vi "Safety_Check.vi"(1 "Adam Loop Count":i32, 2 "Ch Names":string[](array[string]), 3 "Values":dbl[](array[numeric]) format="%.2f") -> (0 "Scan comment":string)   [LabVIEW 2012]
uses:
  ADAM Client/Sub VIs/ADAM Controls/Update_scan_value.ctl
  Anemometry/Anemometry Sub Vis/Globals/Gas_management_global.vi
  ADAM_Global.vi
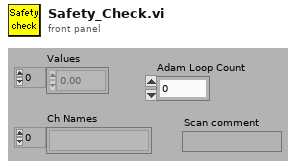
[diagram p1: front panel]
types:
  T1 = cluster{"Channel name":string, "Set value of A to":dbl, "Set value of B to":dbl, "Set value of C to":dbl, "Set value of D to":dbl}
  T2 = typedef "Update_scan_value.ctl" = cluster{"Channel Name":string, "New Value":dbl}
  T3 = enum16{"Append to Global", "Read Global then Clear"}
  T4 = enum16{"On", "Off", "Always On", "Always Off", "Delete"}
  T5 = typedef "LVDateTimeRec.ctl" = cluster{"fractional second":dbl, "second":i32, "minute":i32, "hour":i32, "day of month":i32, "month":i32, "year":i32, "day of week":i32, "day of year":i32, "DST":i32}
  T6 = cluster{"Channel name":string, "Set value of A to":dbl, "Set value of B to":dbl, "Set value of C to":dbl, "Set value of D to":dbl}[]
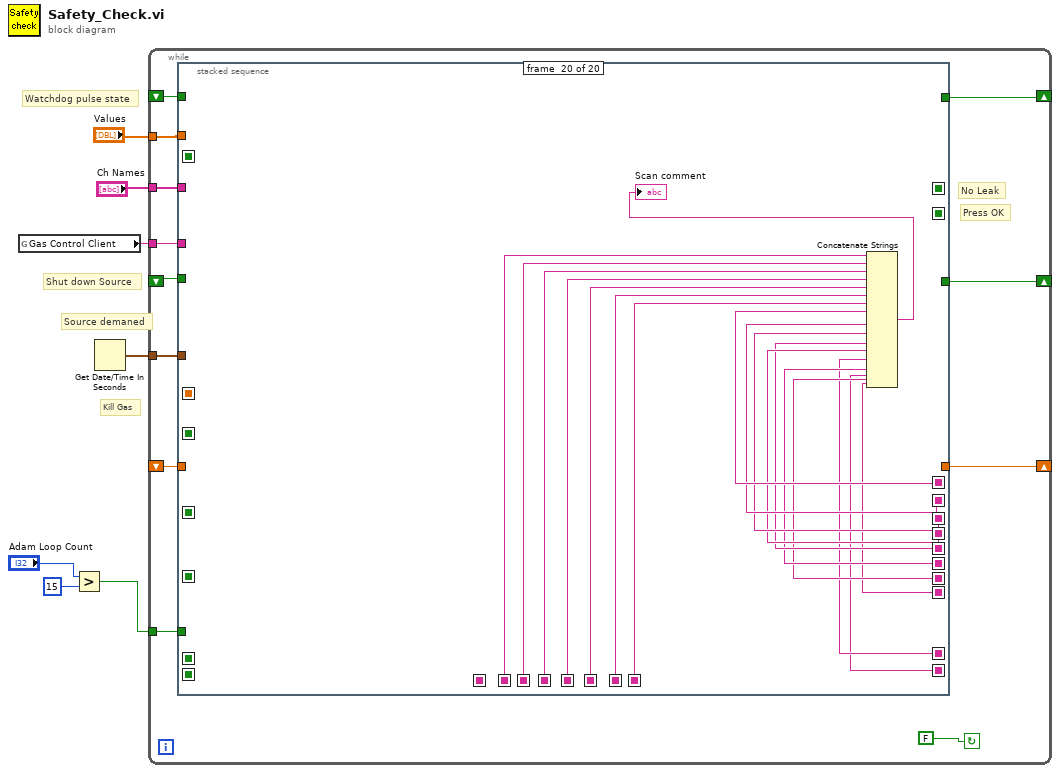
[diagram p0: block diagram]
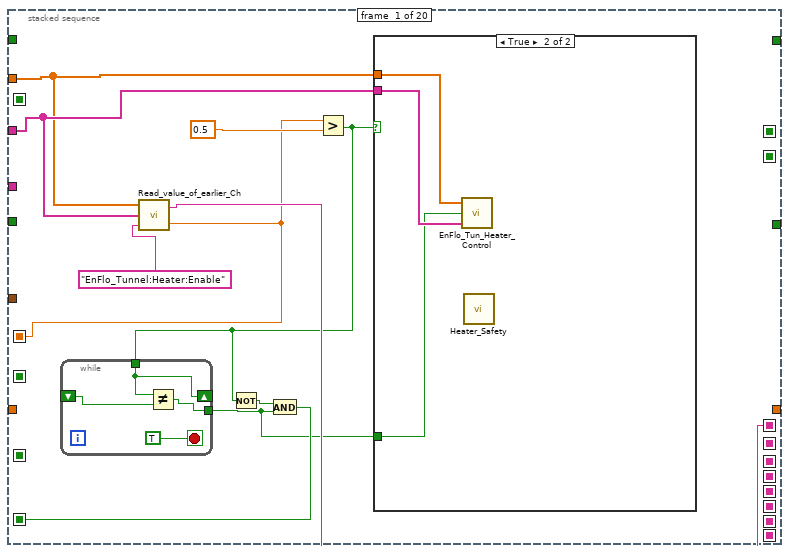
[diagram p2: hidden frame]
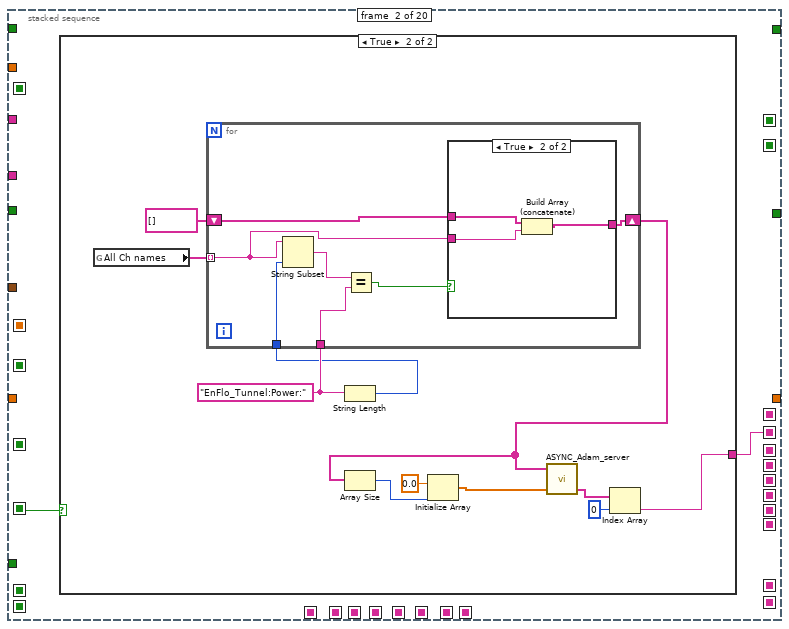
[diagram p4: hidden frame]
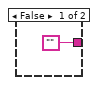
[diagram p5: hidden frame]
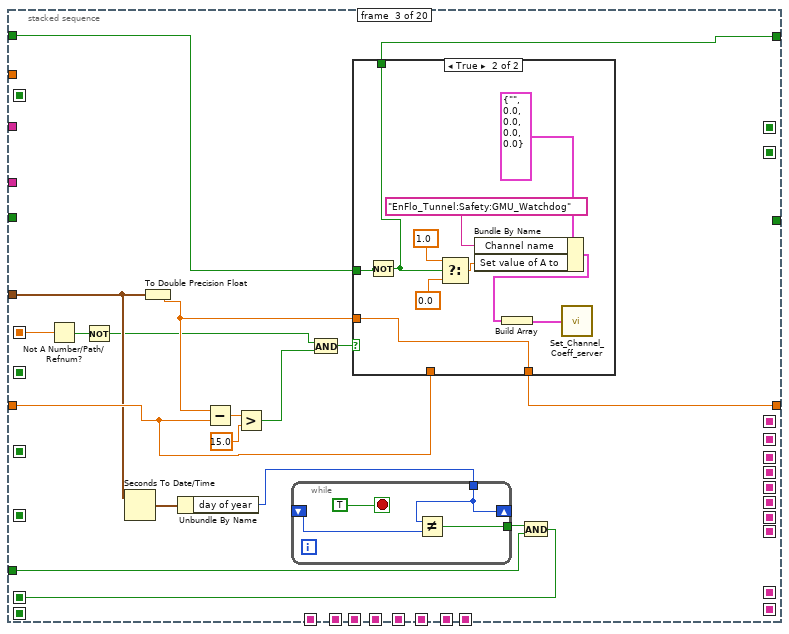
[diagram p7: hidden frame]
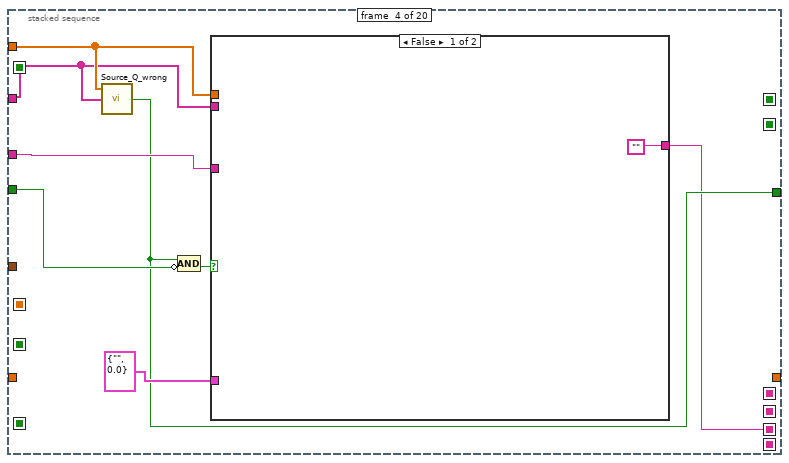
[diagram p9: hidden frame]
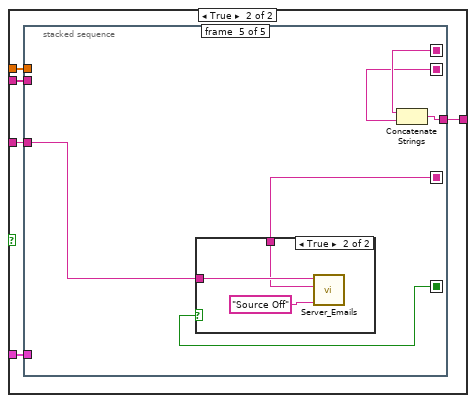
[diagram p10: hidden frame]
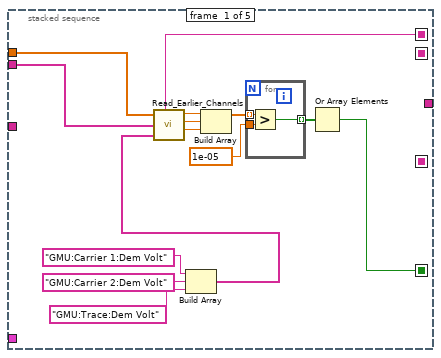
[diagram p11: hidden frame]
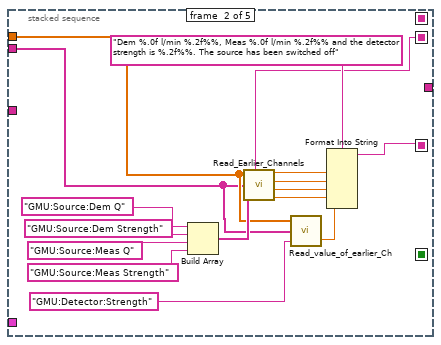
[diagram p12: hidden frame]
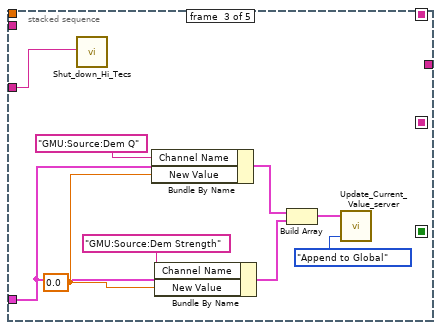
[diagram p13: hidden frame]
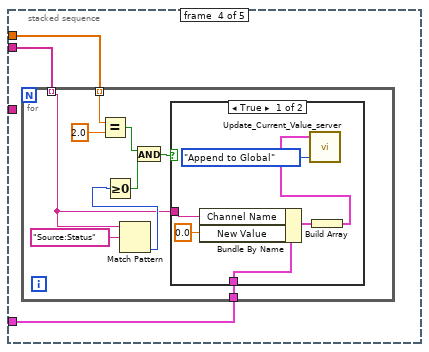
[diagram p14: hidden frame]
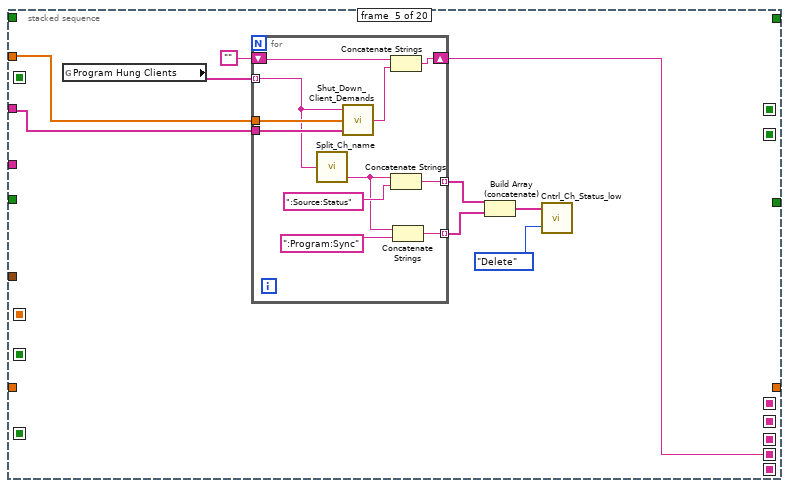
[diagram p17: hidden frame]
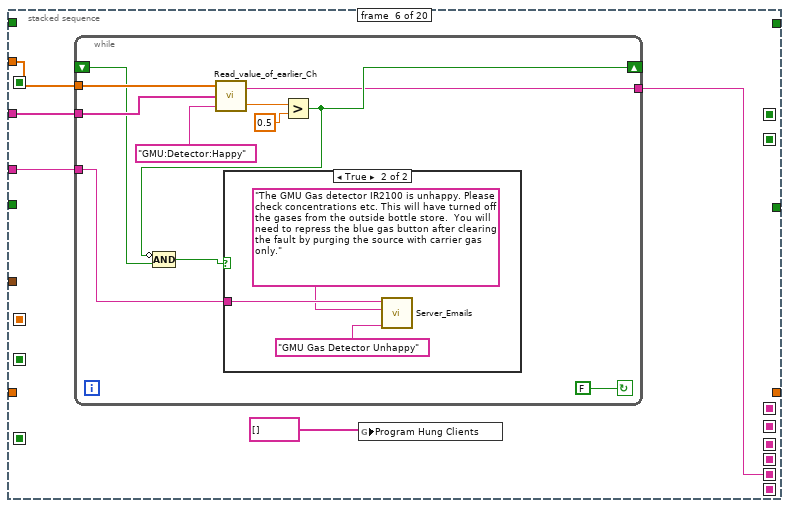
[diagram p18: hidden frame]
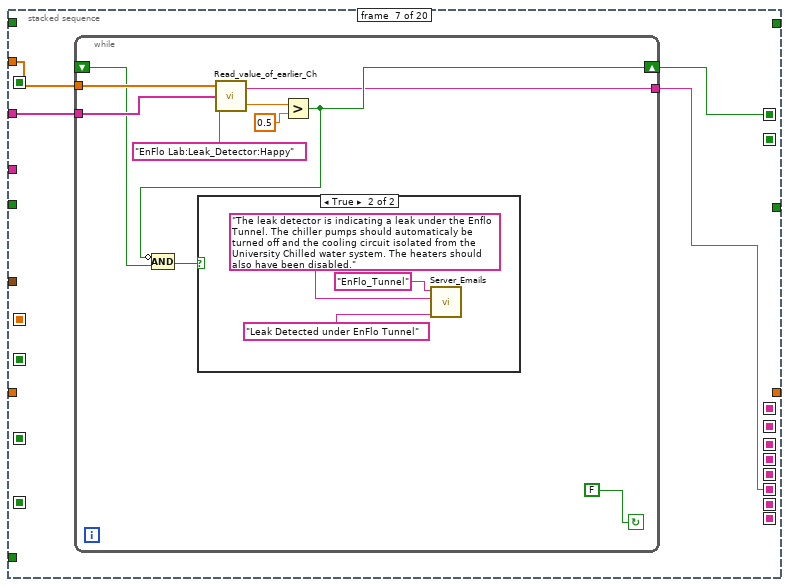
[diagram p20: hidden frame]
diagram:
  # "Shut down Source"
  # "Source demaned"
  # "Watchdog pulse state"
  # "Kill Gas"
  n1 = global read "Gas_management_global.vi" "Gas Control Client"() -> (w5:string)
  n2 = Greater?(x="Adam Loop Count", y=15) -> (0:w2:bool)
  n3 = Get Date/Time In Seconds() -> (seconds since 1Jan1904=w1:timestamp)
  n4 = while {
    shift-left: _ -> [w14]
    shift-right: [w13] -> _
    shift-left: _ -> [w16]
    shift-right: [w15] -> _
    tunnel: w5 -> [w18]
    tunnel: "Ch Names" -> [w19]
    tunnel: "Values" -> [w17]
    shift-right: [w11] -> _
    shift-left: _ -> [w10]
    tunnel: w2 -> [w9]
    tunnel: w1 -> [w8]
    stop <- FALSE continue-if-true
    # "Press OK"
    # "No Leak"
    n5 = stacked-sequence {
      seq-local: [_ _ _ _ _ _ w219 _ _ _ _ _ _ _ _ _ _ _ _ _] -> [_ _ _ _ _ _ _ _ _ _ _ _ w401 _ _ _ _ _ _ _]
      seq-local: [w22 _ _ _ _ _ _ _ _ _ _ _ _ _ _ _ _ _ _ _] -> [_ w38 _ _ _ _ _ _ _ _ _ _ _ _ _ _ _ _ _ _]
      seq-local: [_ _ w68 _ _ _ _ _ _ _ _ _ _ _ _ _ _ _ _ _] -> [_ _ _ _ _ _ _ _ _ _ _ _ _ _ _ _ _ _ _ _]
      seq-local: [_ _ _ _ _ _ _ _ _ _ _ _ _ _ w462 _ _ _ _ _] -> [_ _ _ _ _ _ _ _ _ _ _ _ _ _ _ w478 _ _ _ _]
      seq-local: [_ _ _ _ _ _ _ _ _ _ _ _ _ _ _ w470 _ _ _ _] -> [_ _ _ _ _ _ _ _ _ _ _ _ _ _ _ _ _ _ w602 _]
      seq-local: [w25 _ _ _ _ _ _ _ _ _ _ _ _ _ _ _ _ _ _ _] -> [_ _ _ _ _ _ _ _ _ _ _ _ _ _ _ _ _ _ _ w638]
      seq-local: [_ w37 _ _ _ _ _ _ _ _ _ _ _ _ _ _ _ _ _ _] -> [_ _ _ _ _ _ _ _ _ _ _ _ _ _ _ _ _ _ _ w637]
      seq-local: [_ _ _ w96 _ _ _ _ _ _ _ _ _ _ _ _ _ _ _ _] -> [_ _ _ _ _ _ _ _ _ _ _ _ _ _ _ _ _ _ _ w636]
      seq-local: [_ _ _ _ w179 _ _ _ _ _ _ _ _ _ _ _ _ _ _ _] -> [_ _ _ _ _ _ _ _ _ _ _ _ _ _ _ _ _ _ _ w635]
      seq-local: [_ _ _ _ _ w199 _ _ _ _ _ _ _ _ _ _ _ _ _ _] -> [_ _ _ _ _ _ _ _ _ _ _ _ _ _ _ _ _ _ _ w634]
      seq-local: [_ _ _ _ _ _ w218 _ _ _ _ _ _ _ _ _ _ _ _ _] -> [_ _ _ _ _ _ _ _ _ _ _ _ _ _ _ _ _ _ _ w633]
      seq-local: [_ _ _ _ _ _ _ _ _ w326 _ _ _ _ _ _ _ _ _ _] -> [_ _ _ _ _ _ _ _ _ _ _ _ _ _ _ _ _ _ _ w632]
      seq-local: [_ _ _ _ _ _ _ _ _ _ w358 _ _ _ _ _ _ _ _ _] -> [_ _ _ _ _ _ _ _ _ _ _ _ _ _ _ _ _ _ _ w623]
      seq-local: [_ _ _ _ _ _ _ _ _ _ _ w378 _ _ _ _ _ _ _ _] -> [_ _ _ _ _ _ _ _ _ _ _ _ _ _ _ _ _ _ _ w622]
      seq-local: [_ _ _ _ _ _ _ _ _ _ _ _ w402 _ _ _ _ _ _ _] -> [_ _ _ _ _ _ _ _ _ _ _ _ _ _ _ _ _ _ _ w625]
      seq-local: [_ _ _ _ _ _ _ _ _ _ _ _ _ w429 _ _ _ _ _ _] -> [_ _ _ _ _ _ _ _ _ _ _ _ _ _ _ _ _ _ _ w626]
      seq-local: [_ _ _ _ _ _ _ _ _ _ _ _ _ _ w453 _ _ _ _ _] -> [_ _ _ _ _ _ _ _ _ _ _ _ _ _ _ _ _ _ _ w627]
      seq-local: [_ _ _ _ _ _ _ _ _ _ _ _ _ _ _ w467 _ _ _ _] -> [_ _ _ _ _ _ _ _ _ _ _ _ _ _ _ _ _ _ _ w628]
      seq-local: [_ _ _ _ _ _ _ _ _ _ _ _ _ _ _ _ w535 _ _ _] -> [_ _ _ _ _ _ _ _ _ _ _ _ _ _ _ _ _ _ _ w629]
      seq-local: [_ _ _ _ _ _ _ _ _ _ _ _ _ _ _ _ _ w564 _ _] -> [_ _ _ _ _ _ _ _ _ _ _ _ _ _ _ _ _ _ _ w630]
      seq-local: [_ _ _ _ _ _ _ _ _ _ _ _ _ _ _ _ _ _ w600 _] -> [_ _ _ _ _ _ _ _ _ _ _ _ _ _ _ _ _ _ _ w631]
      seq-local: [w24 _ _ _ _ _ _ _ _ _ _ _ _ _ _ _ _ _ _ _] -> [_ _ w66 _ _ _ _ _ _ _ _ _ _ _ _ _ _ _ _ _]
      seq-local: [_ _ _ _ _ _ _ _ _ _ _ _ _ _ w452 _ _ _ _ _] -> [_ _ _ _ _ _ _ _ _ _ _ _ _ _ _ w466 _ _ _ _]
      seq-local: [_ _ _ _ _ _ _ w237 _ _ _ _ _ _ _ _ _ _ _ _] -> [_ _ _ _ _ _ _ _ _ _ _ _ w400 _ _ _ _ _ _ _]
      seq-local: [_ _ _ _ _ _ _ w236 _ _ _ _ _ _ _ _ _ _ _ _] -> [_ _ _ _ _ _ _ _ _ _ _ _ _ _ _ _ _ _ _ w621]
      seq-local: [_ _ _ _ _ _ _ w235 _ _ _ _ _ _ _ _ _ _ _ _] -> [_ _ _ _ _ _ _ _ w267 _ _ _ _ _ _ _ _ _ _ _]
      seq-local: [_ _ _ _ _ _ _ _ w264 _ _ _ _ _ _ _ _ _ _ _] -> [_ _ _ _ _ _ _ _ _ _ _ _ _ _ _ _ _ _ _ _]
      tunnel: w19 -> [w27 _ _ w98 w186 w201 w220 w238 w265 w327 w359 w380 w403 w435 w458 w479 w540 w567 _ _]
      tunnel: w18 -> [_ _ _ w103 _ w200 _ _ _ _ _ _ _ _ _ _ _ _ _ _]
      tunnel: w17 -> [w26 _ _ w99 w182 w202 w221 w239 w266 w328 w360 w381 w404 w436 w459 w480 w541 w568 _ _]
      tunnel: w16 -> [_ _ w79 _ _ _ _ _ _ _ _ _ _ _ _ _ _ _ _ _]
      tunnel: [_ _ w78 _ _ _ _ _ _ _ _ _ _ _ _ _ _ _ _ _] -> w15
      tunnel: w14 -> [_ _ _ w102 _ _ _ _ _ _ _ _ _ _ _ _ _ _ _ _]
      tunnel: [_ _ _ w97 _ _ _ _ _ _ _ _ _ _ _ _ _ _ _ _] -> w13
      tunnel: [_ _ w77 _ _ _ _ _ _ _ _ _ _ _ _ _ _ _ _ _] -> w11
      tunnel: w10 -> [_ _ w73 _ _ _ _ _ _ _ _ _ _ _ _ _ _ _ _ _]
      tunnel: w9 -> [_ _ w69 _ _ _ _ _ _ _ _ w379 _ _ _ w471 w536 _ w601 _]
      tunnel: w8 -> [_ _ w67 _ _ _ _ _ _ _ _ _ _ _ _ _ _ _ _ _]
      frame #0 {
        n6 = call "Read_value_of_earlier_Ch.vi"("Desired Ch to Read"="EnFlo_Tunnel:Heater:Enable", "Ch names"=w27, "Present scan array"=w26) -> ("Value"=w24:dbl, "Scan comment"=w25:string)  [unwired: 1 in]
        n7 = Greater?(x=w24, y=0.5) -> (0:w23:bool)
        n8 = while {
          shift-right: [w33] -> _
          shift-left: _ -> [w32]
          tunnel: w23 -> [w33]
          tunnel: [w30] -> w20
          stop <- TRUE stop-if-true
          n9 = Not Equal?(x=w33, y=w32) -> (x != y?=w30:bool)
        }
        n10 = Not(x=w23) -> (.not. x?=w21:bool)
        n11 = And(x=w21, y=w20) -> (x .and. y?=w22:bool)
        n12 = case shown="True" w23 {
          tunnel: w26 -> [_ w36]
          tunnel: w27 -> [_ w35]
          tunnel: w20 -> [_ w34]
          frame False {
          }
          frame True {
            n13 = call "EnFlo_Tun_Heater_Control.vi"("Ch Names"=w35, "Heaters Just Enabled"=w34, "Values"=w36) -> ()  [unwired: 1 in]
            n14 = call "Heater_Safety.vi"() -> ()  [unwired: 3 in, 5 out]
          }
        }
      }
      frame #1 {
        n15 = case shown="True" w38 {
          tunnel: ["" w41] -> w37
          frame False {
          }
          frame True {
            w50 = "EnFlo_Tunnel:Power:"
            n16 = global read "ADAM_Global.vi" "All Ch names"() -> (w40:string[])
            n17 = String Length(string=w50) -> (length=w49:i32)
            n18 = for {
              shift-right: [w52] -> w45
              shift-left: string[] [] -> [w53]
              tunnel: w40 -> [w56] mode=indexing
              tunnel: w49 -> [w57]
              tunnel: w50 -> [w54]
              n19 = String Subset(string=w56, length (rest)=w57) -> (substring=w55:string)  [unwired: 1 out]
              n20 = Equal?(x=w55, y=w54) -> (x = y?=w51:bool)
              n21 = case shown="True" w51 {
                tunnel: w56 -> [_ w61]
                tunnel: w53 -> [w58 w59]
                tunnel: [w58 w60] -> w52
                frame False {
                }
                frame True {
                  n22 = Build Array (concatenate)(w59, w61) -> (w60:string[])
                }
              }
            }
            n23 = Array Size(array=w45) -> (size(s)=w46:i32)
            n24 = Initialize Array(0.0 ("element"), w46) -> (w44:dbl[])
            n25 = call "ASYNC_Adam_server.vi"("Values"=w44, "Channel Names"=w45) -> ("Scan Comments"=w43:string[])  [unwired: 1 in, 2 out]
            n26 = Index Array(array=w43, index=0) -> (element=w41:string)
          }
        }
      }
      frame #2 {
        n27 = Not A Number/Path/Refnum?(number/path/refnum=w66) -> (NaN/Path/Refnum?=w65:bool)
        n28 = Not(x=w65) -> (.not. x?=w63:bool)
        n29 = Seconds To Date/Time(time stamp (now)=w67) -> (date time rec=w72:T5)  [unwired: 1 in]
        n30 = To Double Precision Float(number=w67) -> (double precision float=w76:dbl)
        n31 = Unbundle By Name(w72) -> ("day of year"=w71:i32)
        n32 = Subtract(x=w76, y=w73) -> (x-y=w75:dbl)
        n33 = Greater?(x=w75, y=15.0) -> (0:w64:bool)
        n34 = while {
          shift-right: [w83] -> _
          shift-left: _ -> [w82]
          tunnel: w71 -> [w83]
          tunnel: [w81] -> w70
          stop <- TRUE stop-if-true
          n35 = Not Equal?(x=w83, y=w82) -> (x != y?=w81:bool)
        }
        n36 = And(x=w63, y=w64) -> (x .and. y?=w62:bool)
        n37 = case shown="True" w62 {
          tunnel: w79 -> [w84 w88]
          tunnel: [w84 w87] -> w78
          tunnel: [w85 w86] -> w77
          tunnel: w76 -> [_ w86]
          tunnel: w73 -> [w85 _]
          frame False {
          }
          frame True {
            n38 = Not(x=w88) -> (.not. x?=w87:bool)
            n39 = Select(t=1.0 ("Suction"), s=w87, f=0.0 ("Suction")) -> (s? t:f=w91:dbl)
            n40 = Bundle By Name(cluster=T1 {"Channel name"="", "Set value of A to"=0.0, "Set value of B to"=0.0, "Set value of C to"=0.0, "Set value of D to"=0.0}, "Channel name"="EnFlo_Tunnel:Safety:GMU_Watchdog" ("Desired Ch to Read"), "Set value of A to"=w91) -> (w95:T1)
            n41 = Build Array(w95) -> (w90:T6)
            n42 = call "Set_Channel_Coeff_server.vi"("Set Array"=w90) -> ()
          }
        }
        n43 = And(x=w70, y=w69) -> (x .and. y?=w68:bool)
      }
      frame #3 {
        n44 = call "Source_Q_wrong.vi"("Ch Names"=w98, "Values"=w99) -> ("Gas Error?"=w97:bool)  [unwired: 1 out]
        n45 = Compound Arithmetic op=AND(w97, invert w102) -> (w101:bool)
        n46 = case shown="False" w101 {
          tunnel: w103 -> [_ w109]
          tunnel: w99 -> [_ w108]
          tunnel: w98 -> [_ w107]
          tunnel: T2 {"Channel Name"="", "New Value"=0.0} ("Update Scan Value Cluster") -> [_ w106]
          tunnel: ["" w105] -> w96
          frame False {
          }
          frame True {
            n47 = stacked-sequence {
              seq-local: [_ w141 _ _ _] -> [_ _ _ _ w174]
              seq-local: [w111 _ _ _ _] -> [_ _ _ _ w173]
              seq-local: [w110 _ _ _ _] -> [_ _ _ _ w172]
              seq-local: [_ w127 _ _ _] -> [_ _ _ _ w171]
              tunnel: w109 -> [_ _ w144 _ w175]
              tunnel: w108 -> [w121 w131 _ w153 _]
              tunnel: w107 -> [w122 w130 _ w154 _]
              tunnel: w106 -> [_ _ w143 w152 _]
              tunnel: [_ _ _ _ w170] -> w105
              frame #0 {
                n48 = Build Array("GMU:Carrier 1:Dem Volt", "GMU:Carrier 2:Dem Volt", "GMU:Trace:Dem Volt") -> (w123:string[])
                n49 = call "Read_Earlier_Channels.vi"("Present scan array"=w121, "Ch names"=w122, "Desired Channels"=w123) -> ("Scan comments"=w110:string, "Index 0"=w117:dbl, "Index 1"=w116:dbl, "Index 2"=w115:dbl)  [unwired: 2 out]
                n50 = Build Array(w117, w116, w115) -> (w114:dbl[])
                n51 = for {
                  tunnel: w114 -> [w126] mode=indexing
                  tunnel: 1e-05 -> [w125]
                  tunnel: [w124] -> w112 mode=indexing
                  n52 = Greater?(x=w126, y=w125) -> (0:w124:bool)
                }
                n53 = Or Array Elements(Boolean array=w112) -> (logical OR=w111:bool)
              }
              frame #1 {
                n54 = Build Array("GMU:Source:Dem Q", "GMU:Source:Dem Strength", "GMU:Source:Meas Q", "GMU:Source:Meas Strength") -> (w136:string[])
                n55 = call "Read_Earlier_Channels.vi"("Present scan array"=w131, "Ch names"=w130, "Desired Channels"=w136) -> ("Scan comments"=w127:string, "Index 0"=w135:dbl, "Index 1"=w134:dbl, "Index 2"=w133:dbl, "Index 3"=w132:dbl)  [unwired: 1 out]
                n56 = call "Read_value_of_earlier_Ch.vi"("Desired Ch to Read"="GMU:Detector:Strength", "Ch names"=w130, "Present scan array"=w131) -> ("Value"=w128:dbl)  [unwired: 1 in, 1 out]
                n57 = Format Into String(format string="Dem %.0f l/min %.2f%%, Meas %.0f l/min %.2f%% and the detector strength is %.2f%%. The source has been switched off" ("Format String"), w135, w134, w133, w132, w128) -> (resulting string=w141:string)  [unwired: 2 in, 1 out]
              }
              frame #2 {
                w145 = 0.0 ("Bundle Element")
                n58 = call "Shut_down_Hi_Tecs.vi"("Client Name"=w144) -> ()  [unwired: 6 out]
                n59 = Bundle By Name(cluster=w143, "Channel Name"="GMU:Source:Dem Q", "New Value"=w145) -> (w150:T2)
                n60 = Bundle By Name(cluster=w143, "Channel Name"="GMU:Source:Dem Strength", "New Value"=w145) -> (w151:T2)
                n61 = Build Array(w150, w151) -> (w147:T2[])
                n62 = call "Update_Current_Value_server.vi"("Mode"=T3."Append to Global", "Update array in"=w147) -> ()  [unwired: 1 in, 1 out]
              }
              frame #3 {
                n63 = for {
                  tunnel: w154 -> [w155] mode=indexing
                  tunnel: w153 -> [w161] mode=indexing
                  tunnel: w152 -> [w156]
                  n64 = Equal?(x=w161, y=2.0) -> (x = y?=w158:bool)
                  n65 = Match Pattern(string=w155, regular expression="Source:Status") -> (offset past match=w162:i32)  [unwired: 4 out]
                  n66 = Greater Or Equal To 0?(x=w162) -> (x >= 0?=w159:bool)
                  n67 = And(x=w158, y=w159) -> (x .and. y?=w157:bool)
                  n68 = case shown="True" w157 {
                    tunnel: w156 -> [w169 _]
                    tunnel: w155 -> [w168 _]
                    frame True {
                      n69 = Bundle By Name(cluster=w169, "Channel Name"=w168, "New Value"=0.0) -> (w166:T2)
                      n70 = Build Array(w166) -> (w165:T2[])
                      n71 = call "Update_Current_Value_server.vi"("Mode"=T3."Append to Global", "Update array in"=w165) -> ()  [unwired: 1 in, 1 out]
                    }
                    frame False {
                    }
                  }
                }
              }
              frame #4 {
                n72 = case shown="True" w173 {
                  tunnel: w175 -> [_ w178]
                  tunnel: w174 -> [_ w177]
                  frame False {
                  }
                  frame True {
                    n73 = call "Server_Emails.vi"("Client Name Contains"=w178, "Message"=w177, "Subject"="Source Off") -> ()  [unwired: 2 in, 3 out]
                  }
                }
                n74 = Concatenate Strings(w172, w171) -> (w170:string)
              }
            }
          }
        }
      }
      frame #4 {
        n75 = global read "ADAM_Global.vi" "Program Hung Clients"() -> (w187:string[])
        n76 = for {
          tunnel: w187 -> [w196] mode=indexing
          tunnel: w182 -> [w198]
          tunnel: w186 -> [w197]
          tunnel: [w194] -> w185 mode=indexing
          tunnel: [w191] -> w184 mode=indexing
          shift-right: [w189] -> w179
          shift-left: "" -> [w190]
          n77 = call "Split_Ch_name.vi"("Ch name"=w196) -> ("Low level"=w193:string)  [unwired: 2 out]
          n78 = call "Shut_Down_Client_Demands.vi"("Ch Names"=w197, "Values"=w198, "Client Name"=w196) -> ("Comments"=w188:string)
          n79 = Concatenate Strings(w190, w188) -> (w189:string)
          n80 = Concatenate Strings(w193, ":Source:Status") -> (w194:string)
          n81 = Concatenate Strings(w193, ":Program:Sync") -> (w191:string)
        }
        n82 = Build Array (concatenate)(w185, w184) -> (w183:string[])
        n83 = call "Cntrl_Ch_Status_low.vi"("Mode"=T4."Delete", "Channel names"=w183) -> ()  [unwired: 1 out]
      }
      frame #5 {
        n84 = while {
          tunnel: w202 -> [w214]
          tunnel: w201 -> [w213]
          shift-right: [w208] -> _
          shift-left: _ -> [w209]
          tunnel: w200 -> [w206]
          tunnel: [w204] -> w199
          stop <- FALSE continue-if-true
          n85 = call "Read_value_of_earlier_Ch.vi"("Desired Ch to Read"="GMU:Detector:Happy", "Ch names"=w213, "Present scan array"=w214) -> ("Value"=w211:dbl, "Scan comment"=w204:string)  [unwired: 1 in]
          n86 = Greater?(x=w211, y=0.5) -> (0:w208:bool)
          n87 = Compound Arithmetic op=AND(invert w208, w209) -> (w207:bool)
          n88 = case shown="True" w207 {
            tunnel: w206 -> [_ w216]
            frame False {
            }
            frame True {
              n89 = call "Server_Emails.vi"("Client Name Contains"=w216, "Message"="The GMU Gas detector IR2100 is unhappy. Please check concentrations etc. This will have turned off the gases from the outside bottle store.  You will need to repress the blue gas button after clearing the fault by purging the source with carrier gas only.", "Subject"="GMU Gas Detector Unhappy") -> ()  [unwired: 2 in, 3 out]
            }
          }
        }
        n90 = global write "ADAM_Global.vi" "Program Hung Clients"(string[] [] ("Program Hung Clients")) -> ()
      }
      frame #6 {
        n91 = while {
          tunnel: w221 -> [w231]
          tunnel: w220 -> [w230]
          shift-right: [w225] -> w219
          shift-left: _ -> [w226]
          tunnel: [w222] -> w218
          stop <- FALSE continue-if-true
          n92 = call "Read_value_of_earlier_Ch.vi"("Desired Ch to Read"="EnFlo Lab:Leak_Detector:Happy", "Ch names"=w230, "Present scan array"=w231) -> ("Value"=w228:dbl, "Scan comment"=w222:string)  [unwired: 1 in]
          n93 = Greater?(x=w228, y=0.5) -> (0:w225:bool)
          n94 = Compound Arithmetic op=AND(invert w225, w226) -> (w224:bool)
          n95 = case shown="True" w224 {
            frame False {
            }
            frame True {
              n96 = call "Server_Emails.vi"("Client Name Contains"="EnFlo_Tunnel", "Message"="The leak detector is indicating a leak under the Enflo Tunnel. The chiller pumps should automaticaly be turned off and the cooling circuit isolated from the  University Chilled water system. The heaters should also have been disabled.", "Subject"="Leak Detected under EnFlo Tunnel") -> ()  [unwired: 2 in, 3 out]
            }
          }
        }
      }
      frame #7 {
        n97 = while {
          tunnel: w239 -> [w245]
          tunnel: w238 -> [w244]
          shift-right: [w256] -> w237
          shift-left: _ -> [w257]
          tunnel: [w248] -> w236
          tunnel: [w240] -> w235
          stop <- FALSE continue-if-true
          n98 = call "Read_value_of_earlier_Ch.vi"("Desired Ch to Read"="EnFlo_Tunnel:Chiller_Pump:Enable", "Ch names"=w244, "Present scan array"=w245) -> ("Value"=w251:dbl, "Scan comment"=w249:string)  [unwired: 1 in]
          n99 = call "Read_value_of_earlier_Ch.vi"("Desired Ch to Read"="EnFlo_Tunnel:Chilled Water:Pressure_OK", "Ch names"=w244, "Present scan array"=w245) -> ("Value"=w259:dbl, "Scan comment"=w250:string)  [unwired: 1 in]
          n100 = call "Read_value_of_earlier_Ch.vi"("Desired Ch to Read"="EnFlo_Tunnel:Chiller_Pump:Running", "Ch names"=w244, "Present scan array"=w245) -> ("Value"=w242:dbl, "Scan comment"=w241:string)  [unwired: 1 in]
          n101 = Greater?(x=w259, y=0.5) -> (0:w256:bool)
          n102 = Greater?(x=w251, y=0.5) -> (0:w247:bool)
          n103 = Compound Arithmetic op=AND(invert w256, w257, w247) -> (w255:bool)
          n104 = case shown="True" w255 {
            frame False {
            }
            frame True {
              n105 = call "Server_Emails.vi"("Client Name Contains"="EnFlo_Tunnel", "Message"="The pressure in the chilled water  for the Enflo Tunnel has tripped the system. The chiller pumps should automaticaly be turned off and the cooling circuit isolated from the  University Chilled water system. The heaters should also have been disabled.", "Subject"="EnFlo Chilled Water Overpressure Trip") -> ()  [unwired: 2 in, 3 out]
            }
          }
          n106 = Greater?(x=w242, y=0.5) -> (0:w240:bool)
          n107 = Concatenate Strings(w249, w250, w241) -> (w248:string)
        }
      }
      frame #8 {
        n108 = case shown="True" w267 {
          tunnel: w266 -> [_ w296]
          tunnel: w265 -> [_ w295]
          tunnel: ["" w269] -> w264
          frame False {
          }
          frame True {
            w274 = "EnFlo_Tunnel:Chilled Water:Motor_Dem_Voltage"
            # "EnFlo_Tunnel:Chiller_Pump:Running"
            n109 = call "Read_value_of_earlier_Ch.vi"("Desired Ch to Read"="EnFlo_Tunnel:Chilled Water:Pressure_supply (Bar)", "Ch names"=w295, "Present scan array"=w296) -> ("Value"=w281:dbl, "Scan comment"=w273:string)  [unwired: 1 in]
            n110 = call "Read_value_of_earlier_Ch.vi"("Desired Ch to Read"="EnFlo_Tunnel:Chilled Water:Pressure_return (Bar)", "Ch names"=w295, "Present scan array"=w296) -> ("Value"=w291:dbl, "Scan comment"=w272:string)  [unwired: 1 in]
            n111 = call "Read_value_of_earlier_Ch.vi"("Desired Ch to Read"="EnFlo_Tunnel:Chilled Water:Desired_Delta_P", "Ch names"=w295, "Present scan array"=w296) -> ("Value"=w289:dbl, "Scan comment"=w271:string)  [unwired: 1 in]
            n112 = call "Read_value_of_earlier_Ch.vi"("Desired Ch to Read"=w274, "Ch names"=w295, "Present scan array"=w296) -> ("Value"=w279:dbl, "Scan comment"=w270:string)  [unwired: 1 in]
            n113 = Subtract(x=w281, y=w291) -> (x-y=w290:dbl)
            n114 = Subtract(x=w290, y=w289) -> (x-y=w277:dbl)
            n115 = Concatenate Strings(w273, w272, w271, w270) -> (w269:string)
            n116 = In Range and Coerce(upper limit=0.1 ("lower limit"), x=w277, lower limit=-0.1) -> (In Range?=w284:bool)  [unwired: 1 out]
            n117 = Less?(x=w281, y=3.9) -> (x < y?=w285:bool)
            n118 = Select(t=w284, s=w285, f=TRUE) -> (s? t:f=w278:bool)
            n119 = Less?(x=w281, y=4.0) -> (x < y?=w280:bool)
            n120 = case shown="True" w280 {
              tunnel: w279 -> [w307 w310]
              tunnel: w278 -> [_ w312]
              tunnel: w277 -> [_ w311]
              tunnel: [TRUE w309] -> w276
              tunnel: [w304 w308] -> w275
              frame False {
                n121 = Subtract(x=w307, y=0.2) -> (x-y=w304:dbl)
              }
              frame True {
                n122 = case shown="False" w312 {
                  tunnel: w311 -> [w317 _]
                  tunnel: w310 -> [w316 w324]
                  tunnel: [TRUE FALSE] -> w309
                  tunnel: [w314 w324] -> w308
                  frame False {
                    n123 = Greater Than 0?(x=w317) -> (x > 0?=w315:bool)
                    n124 = case shown="False" w315 {
                      tunnel: w316 -> [w319 w322]
                      tunnel: [w318 w321] -> w314
                      frame True {
                        n125 = Subtract(x=w319, y=0.1) -> (x-y=w318:dbl)
                      }
                      frame False {
                        n126 = Add(x=w322, y=0.1) -> (x+y=w321:dbl)
                      }
                    }
                  }
                  frame True {
                  }
                }
              }
            }
            n127 = case shown="True" w276 {
              tunnel: w275 -> [_ w298]
              tunnel: w274 -> [_ w301]
              frame False {
              }
              frame True {
                n128 = In Range and Coerce(upper limit=10.0, x=w298, lower limit=0.0) -> (coerced(x)=w297:dbl)  [unwired: 1 out]
                n129 = Build Array(w301) -> (w302:string[])
                n130 = Build Array(w297) -> (w303:dbl[])
                n131 = call "ASYNC_Adam_server.vi"("Values"=w303, "Channel Names"=w302) -> ()  [unwired: 1 in, 3 out]
              }
            }
          }
        }
      }
      frame #9 {
        n132 = while {
          tunnel: w328 -> [w344]
          tunnel: w327 -> [w343]
          shift-right: [w337] -> _
          shift-left: _ -> [w333]
          tunnel: [w329] -> w326
          stop <- FALSE continue-if-true
          w335 = 60.0 ("y")
          n133 = Decrement(x=w335) -> (x-1=w336:dbl)
          n134 = Select(t=w336, s=w333, f=w335) -> (s? t:f=w334:dbl)
          n135 = call "Read_value_of_earlier_Ch.vi"("Desired Ch to Read"="EnFlo_Tunnel:Chilled Water:Motor1 Temp", "Ch names"=w343, "Present scan array"=w344) -> ("Value"=w351:dbl, "Scan comment"=w331:string)  [unwired: 1 in]
          n136 = call "Read_value_of_earlier_Ch.vi"("Desired Ch to Read"="EnFlo_Tunnel:Chilled Water:Motor2 Temp", "Ch names"=w343, "Present scan array"=w344) -> ("Value"=w348:dbl, "Scan comment"=w330:string)  [unwired: 1 in]
          n137 = Greater?(x=w351, y=w334) -> (0:w345:bool)
          n138 = Greater?(x=w348, y=w334) -> (0:w346:bool)
          n139 = Or(x=w345, y=w346) -> (x .or. y?=w339:bool)
          n140 = call "Read_value_of_earlier_Ch.vi"("Desired Ch to Read"="EnFlo_Tunnel:Chiller_Pump:Enable", "Ch names"=w343, "Present scan array"=w344) -> ("Value"=w341:dbl, "Scan comment"=w332:string)  [unwired: 1 in]
          n141 = Greater?(x=w341, y=0.5) -> (0:w338:bool)
          n142 = And(x=w338, y=w339) -> (x .and. y?=w337:bool)
          n143 = Compound Arithmetic op=AND(w337, invert w333) -> (w350:bool)
          n144 = case shown="False" w350 {
            tunnel: w335 -> [_ w354]
            frame False {
            }
            frame True {
              n145 = Format Into String(format string="The Chilled Water Motor Temp is greater than %.0f deg C." ("Message"), w354) -> (resulting string=w353:string)  [unwired: 2 in, 1 out]
              n146 = call "Server_Emails.vi"("Client Name Contains"="EnFlo_Tunnel", "Message"=w353, "Subject"="Chilled Water Motor Temp") -> ()  [unwired: 2 in, 3 out]
            }
          }
          n147 = Concatenate Strings(w332, w331, w330) -> (w329:string)
        }
      }
      frame #10 {
        n148 = while {
          tunnel: w360 -> [w374]
          tunnel: w359 -> [w373]
          shift-right: [w362] -> _
          shift-left: _ -> [w368]
          shift-left: _ -> [w367]
          shift-left: _ -> [w366]
          tunnel: [w361] -> w358
          stop <- FALSE continue-if-true
          n149 = call "Read_value_of_earlier_Ch.vi"("Desired Ch to Read"="FFID:System:Enable", "Ch names"=w373, "Present scan array"=w374) -> ("Value"=w369:dbl, "Scan comment"=w361:string)  [unwired: 1 in]
          n150 = Greater?(x=w369, y=0.5) -> (0:w362:bool)
          n151 = Compound Arithmetic op=AND(w362, w368, invert w367, invert w366) -> (w364:bool)
          n152 = Compound Arithmetic op=AND(invert w362, invert w368, w367, w366) -> (w365:bool)
          n153 = Or(x=w364, y=w365) -> (x .or. y?=w363:bool)
          n154 = case shown="True" w363 {
            tunnel: w369 -> [_ w375]
            tunnel: w362 -> [_ _]
            frame False {
            }
            frame True {
              n155 = Build Array(w375) -> (w377:dbl[])
              n156 = call "ASYNC_Adam_server.vi"("Values"=w377, "Channel Names"=string[] ["GMU:Gas:Enable"]) -> ()  [unwired: 1 in, 3 out]
            }
          }
        }
      }
      frame #11 {
        # "Resetting A Tunnel speed to zero if the drive in turned off\nso that the belts do not slip when the tunnel is turned on again."
        n157 = while {
          tunnel: w381 -> [w394]
          tunnel: w380 -> [w393]
          shift-right: [w385] -> _
          shift-left: _ -> [w388]
          shift-left: _ -> [w387]
          shift-left: _ -> [w386]
          tunnel: w379 -> [w384]
          tunnel: [w382] -> w378
          stop <- FALSE continue-if-true
          n158 = call "Read_value_of_earlier_Ch.vi"("Desired Ch to Read"="A_Tunnel:Motor:Enable", "Ch names"=w393, "Present scan array"=w394) -> ("Value"=w389:dbl, "Scan comment"=w382:string)  [unwired: 1 in]
          n159 = Less?(x=w389, y=0.5) -> (x < y?=w385:bool)
          n160 = Compound Arithmetic op=AND(w385, w388, invert w387, invert w386, w384) -> (w383:bool)
          n161 = case shown="True" w383 {
            tunnel: w385 -> [_ _]
            frame False {
            }
            frame True {
              w397 = string[] ["A_Tunnel:Speed:Dem Velocity", "A_Tunnel:Speed:Dem Voltage"] ("Channel Names")
              n162 = Array Size(array=w397) -> (size(s)=w398:i32)
              n163 = Initialize Array(0.0 ("element"), w398) -> (w396:dbl[])
              n164 = call "ASYNC_Adam_server.vi"("Values"=w396, "Channel Names"=w397) -> ()  [unwired: 1 in, 3 out]
            }
          }
        }
      }
      frame #12 {
        n165 = And(x=w400, y=w401) -> (x .and. y?=w399:bool)
        n166 = case shown="False" w399 {
          tunnel: w404 -> [w409 _]
          tunnel: w403 -> [w408 _]
          tunnel: [w405 ""] -> w402
          frame False {
            n167 = for {
              tunnel: w409 -> [w419]
              tunnel: w408 -> [w418]
              tunnel: string[] ["EnFlo_Tunnel:Heater:Enable", "EnFlo_Tunnel:Chiller_Pump:Enable", "EnFlo_Tunnel:Tap_Water:Enable"] ("Ch Names") -> [w414] mode=indexing
              shift-right: [w412] -> w405
              shift-left: "" -> [w413]
              n168 = call "Read_value_of_earlier_Ch.vi"("Desired Ch to Read"=w414, "Ch names"=w418, "Present scan array"=w419) -> ("Value"=w416:dbl, "Scan comment"=w411:string)  [unwired: 1 in]
              n169 = Greater?(x=w416, y=0.5) -> (0:w415:bool)
              n170 = case shown="True" w415 {
                tunnel: w414 -> [_ w424]
                tunnel: ["" w421] -> w410
                frame False {
                }
                frame True {
                  n171 = Build Array(w424) -> (w427:string[])
                  n172 = Build Array(0.0) -> (w426:dbl[])
                  n173 = call "ASYNC_Adam_server.vi"("Values"=w426, "Channel Names"=w427) -> ("Scan Comments"=w422:string[])  [unwired: 1 in, 2 out]
                  n174 = Index Array(array=w422, index=0) -> (element=w421:string)
                }
              }
              n175 = Concatenate Strings(w413, w411, w410) -> (w412:string)
            }
          }
          frame True {
          }
        }
      }
      frame #13 {
        w437 = "EnFlo_Tunnel:Heater:Enable" ("Ch Name")
        n176 = call "Read_value_of_earlier_Ch.vi"("Desired Ch to Read"=w437, "Ch names"=w435, "Present scan array"=w436) -> ("Value"=w442:dbl, "Scan comment"=w431:string)  [unwired: 1 in]
        n177 = call "Read_value_of_earlier_Ch.vi"("Desired Ch to Read"="EnFlo_Tunnel:Reference:Velocity", "Ch names"=w435, "Present scan array"=w436) -> ("Value"=w439:dbl, "Scan comment"=w430:string)  [unwired: 1 in]
        n178 = Greater?(x=w442, y=0.5) -> (0:w434:bool)
        n179 = Less?(x=w439, y=0.25) -> (x < y?=w438:bool)
        n180 = And(x=w434, y=w438) -> (x .and. y?=w433:bool)
        n181 = case shown="True" w433 {
          tunnel: w437 -> [_ w448]
          tunnel: ["" w445] -> w432
          frame False {
          }
          frame True {
            n182 = Build Array(w448) -> (w451:string[])
            n183 = Build Array(0.0) -> (w450:dbl[])
            n184 = call "ASYNC_Adam_server.vi"("Values"=w450, "Channel Names"=w451) -> ("Scan Comments"=w446:string[])  [unwired: 1 in, 2 out]
            n185 = Index Array(array=w446, index=0) -> (element=w445:string)
          }
        }
        n186 = Concatenate Strings(w431, w430, w432) -> (w429:string)
      }
      frame #14 {
        n187 = call "Read_value_of_earlier_Ch.vi"("Desired Ch to Read"="EnFlo_Tunnel:Chiller_Pump:Running", "Ch names"=w458, "Present scan array"=w459) -> ("Value"=w460:dbl, "Scan comment"=w455:string)  [unwired: 1 in]
        n188 = call "Read_value_of_earlier_Ch.vi"("Desired Ch to Read"="EnFlo_Tunnel:Reference:Velocity", "Ch names"=w458, "Present scan array"=w459) -> ("Value"=w456:dbl, "Scan comment"=w454:string)  [unwired: 1 in]
        n189 = Greater?(x=w456, y=0.4) -> (0:w464:bool)
        n190 = Greater?(x=w460, y=0.5) -> (0:w452:bool)
        n191 = Compound Arithmetic op=AND(w452, w464) -> (w462:bool)
        n192 = Concatenate Strings(w455, w454) -> (w453:string)
      }
      frame #15 {
        w476 = "EnFlo_Tunnel:Heat_Ex_Div_Valve:Dem Pos"
        n193 = case shown="True" w478 {
          tunnel: w480 -> [_ w518]
          tunnel: w479 -> [_ w519]
          tunnel: w476 -> [_ w522]
          tunnel: [0.0 ("upper limit") w528] -> w472
          tunnel: ["" w513] -> w469
          frame False {
          }
          frame True {
            n194 = call "Read_value_of_earlier_Ch.vi"("Desired Ch to Read"="EnFlo_Tunnel:Exit Duct:Dem Temp", "Ch names"=w519, "Present scan array"=w518) -> ("Value"=w527:dbl, "Scan comment"=w517:string)  [unwired: 1 in]
            n195 = call "Read_value_of_earlier_Ch.vi"("Desired Ch to Read"="EnFlo_Tunnel:Exit Duct Top:Temp", "Ch names"=w519, "Present scan array"=w518) -> ("Value"=w523:dbl, "Scan comment"=w516:string)  [unwired: 1 in]
            n196 = call "Read_value_of_earlier_Ch.vi"("Desired Ch to Read"="EnFlo_Tunnel:Exit Duct:Temp", "Ch names"=w519, "Present scan array"=w518) -> ("Value"=w524:dbl, "Scan comment"=w515:string)  [unwired: 1 in]
            n197 = call "Read_value_of_earlier_Ch.vi"("Desired Ch to Read"=w522, "Ch names"=w519, "Present scan array"=w518) -> ("Value"=w525:dbl, "Scan comment"=w514:string)  [unwired: 1 in]
            n198 = Add(x=w523, y=w524) -> (x+y=w532:dbl)
            n199 = Divide(x=w532, y=2.0) -> (x/y=w534:dbl)
            n200 = Concatenate Strings(w517, w516, w515, w514) -> (w513:string)
            n201 = call "Back_End_Chiller_PID.vi"("Present Value"=w534, "Previous Control Sum"=w525, "Setpoint"=w527) -> ("Dem Output"=w531:dbl)
            n202 = In Range and Coerce(upper limit=100.0, x=w531, lower limit=0.0) -> (coerced(x)=w528:dbl)  [unwired: 1 out]
          }
        }
        n203 = while {
          shift-right: [w510] -> w477
          shift-left: _ -> [_]
          tunnel: w466 -> [w510]
          shift-left: _ -> [_]
          shift-left: _ -> [_]
          shift-left: _ -> [_]
          shift-left: _ -> [_]
          shift-left: _ -> [_]
          shift-left: _ -> [_]
          shift-left: _ -> [_]
          shift-left: _ -> [_]
          shift-left: _ -> [_]
          shift-left: _ -> [_]
          shift-left: _ -> [_]
          shift-left: _ -> [_]
          shift-left: _ -> [_]
          shift-left: _ -> [_]
          shift-left: _ -> [_]
          shift-left: _ -> [_]
          shift-left: _ -> [w509]
          tunnel: [w509] -> w475
          stop <- TRUE stop-if-true
        }
        n204 = And(x=w477, y=w475) -> (x .and. y?=w474:bool)
        n205 = case shown="False" w474 {
          tunnel: [w482 w493] -> w473
          tunnel: w472 -> [_ w493]
          tunnel: [w481 FALSE] -> w470
          frame False {
            # "Exercise valve once a week"
            n206 = Seconds To Date/Time() -> (date time rec=w483:T5)  [unwired: 2 out]
            n207 = Unbundle By Name(w483) -> ("day of week"=w488:i32, "hour"=w486:i32)
            n208 = Less?(x=w486, y=3) -> (x < y?=w491:bool)
            n209 = Equal?(x=7, y=w488) -> (x = y?=w490:bool)
            n210 = And(x=w490, y=w491) -> (x .and. y?=w481:bool)
            n211 = Select(t=100.0, s=w481, f=0.0) -> (s? t:f=w482:dbl)
          }
          frame True {
          }
        }
        n212 = while {
          shift-right: [w499] -> _
          shift-left: _ -> [w500]
          tunnel: w473 -> [w499]
          tunnel: w476 -> [w501]
          tunnel: w471 -> [w496]
          tunnel: [w494] -> w468
          stop <- TRUE stop-if-true
          n213 = Not Equal?(x=w499, y=w500) -> (x != y?=w497:bool)
          n214 = Compound Arithmetic op=OR(w497, invert w496) -> (w495:bool)
          n215 = Build Array(w501) -> (w502:string[])
          n216 = Build Array(w499) -> (w503:dbl[])
          n217 = case shown="False" w495 {
            tunnel: w503 -> [_ w507]
            tunnel: w502 -> [_ w506]
            tunnel: [string[] [] ("Scan Comments") w505] -> w494
            frame False {
            }
            frame True {
              n218 = call "ASYNC_Adam_server.vi"("Values"=w507, "Channel Names"=w506) -> ("Scan Comments"=w505:string[])  [unwired: 1 in, 2 out]
            }
          }
        }
        n219 = Concatenate Strings(w469, w468) -> (w467:string)
      }
      frame #16 {
        n220 = Search 1D Array(1D array=w540, element="Status:of:EnFlo_Tunnel") -> (index of element=w543:i32)  [unwired: 1 out]
        n221 = Index Array(array=w541, index=w543) -> (element=w539:dbl)
        n222 = case shown="0, Default" w539 {
          tunnel: [0.0 1.0 1.0 1.0] -> w538
          frame 0, Default {
          }
          frame 1 {
          }
          frame 2 {
          }
          frame 3 {
          }
        }
        n223 = while {
          shift-right: [w553] -> _
          shift-left: _ -> [w554]
          tunnel: w538 -> [w553]
          tunnel: "EnFlo_Tunnel:Warning_Cone:Enable" -> [w555]
          tunnel: w536 -> [w550]
          tunnel: [w548] -> w535
          stop <- TRUE stop-if-true
          n224 = Not Equal?(x=w553, y=w554) -> (x != y?=w551:bool)
          n225 = Build Array(w555) -> (w556:string[])
          n226 = Build Array(w553) -> (w557:dbl[])
          n227 = Compound Arithmetic op=OR(w551, invert w550) -> (w549:bool)
          n228 = case shown="True" w549 {
            tunnel: w557 -> [_ w563]
            tunnel: w556 -> [_ w562]
            tunnel: ["" w559] -> w548
            frame False {
            }
            frame True {
              n229 = call "ASYNC_Adam_server.vi"("Values"=w563, "Channel Names"=w562) -> ("Scan Comments"=w560:string[])  [unwired: 1 in, 2 out]
              n230 = Index Array(array=w560, index=0) -> (element=w559:string)
            }
          }
        }
      }
      frame #17 {
        # "To automatically control the request for the University Stall chiller to run."
        n231 = while {
          tunnel: w568 -> [w576]
          tunnel: w567 -> [w577]
          shift-right: [w571] -> _
          shift-left: _ -> [w586]
          shift-left: _ -> [w585]
          shift-left: _ -> [w584]
          tunnel: [w570] -> w566
          tunnel: [w569] -> w565
          stop <- FALSE continue-if-true
          n232 = Build Array("EnFlo_Tunnel:Chiller_Pump:Enable" ("Desired Ch to Read"), "Aero_Tunnel:Cooling_Pump:Enable" ("Desired Ch to Read")) -> (w578:string[])
          n233 = call "Read_Earlier_Channels.vi"("Present scan array"=w576, "Ch names"=w577, "Desired Channels"=w578) -> ("Scan comments"=w569:string, "Index 0"=w575:dbl, "Index 1"=w574:dbl)  [unwired: 3 out]
          n234 = Build Array(w575, w574) -> (w573:dbl[])
          n235 = Greater?(x=w573, y=0.5) -> (0:w572:bool[])
          n236 = Or Array Elements(Boolean array=w572) -> (logical OR=w571:bool)
          n237 = Compound Arithmetic op=AND(w571, w586, invert w585, invert w584) -> (w582:bool)
          n238 = Compound Arithmetic op=AND(invert w571, invert w586, w585, w584) -> (w583:bool)
          n239 = Or(x=w582, y=w583) -> (x .or. y?=w581:bool)
          n240 = case shown="True" w581 {
            tunnel: w571 -> [_ w595]
            tunnel: [string[] [] ("Scan Comments") w590] -> w570
            frame False {
            }
            frame True {
              n241 = case shown="False" w595 {
                tunnel: [string[] ["University:Chilled Water:Requested"] ("Channel Names") string[] ["University:Chilled Water:Requested"] ("Channel Names")] -> w594
                tunnel: [1.0 ("y") 0.0 ("y")] -> w591
                frame True {
                }
                frame False {
                }
              }
              n242 = Array Size(array=w594) -> (size(s)=w592:i32)
              n243 = Initialize Array(w591, w592) -> (w593:dbl[])
              n244 = call "ASYNC_Adam_server.vi"("Values"=w593, "Channel Names"=w594) -> ("Scan Comments"=w590:string[])  [unwired: 1 in, 2 out]
            }
          }
        }
        n245 = Concatenate Strings(w566, w565) -> (w564:string)
      }
      frame #18 {
        # "Exercise the floor cooling valve once a week"
        n246 = while {
          shift-right: [w604] -> _
          shift-left: _ -> [w609]
          tunnel: w602 -> [w604]
          tunnel: w601 -> [w606]
          tunnel: [w603] -> w600
          stop <- TRUE stop-if-true
          n247 = Not Equal?(x=w604, y=w609) -> (x != y?=w607:bool)
          n248 = Compound Arithmetic op=AND(w607, w606) -> (w605:bool)
          n249 = case shown="True" w605 {
            tunnel: w604 -> [_ w616]
            tunnel: ["" w611] -> w603
            frame False {
            }
            frame True {
              n250 = Select(t=1.0, s=w616, f=0.0) -> (s? t:f=w617:dbl)
              n251 = Build Array(w617) -> (w620:dbl[])
              n252 = Build Array("EnFlo_Tunnel:Floor_Cooling:Enable") -> (w619:string[])
              n253 = call "ASYNC_Adam_server.vi"("Values"=w620, "Channel Names"=w619) -> ("Scan Comments"=w612:string[])  [unwired: 1 in, 2 out]
              n254 = Index Array(array=w612, index=0) -> (element=w611:string)
            }
          }
        }
      }
      frame #19 {
        n255 = Concatenate Strings(w625, w626, w627, w628, w629, w630, w631, w638, w637, w636, w635, w634, w633, w632, w623, w622, w621) -> (→"Scan comment":string)
      }
    }
  }
